vi "SetQuestionableInstrumentSMURegister.vi"(7 "SMU":T2, 8 "Error In":errorcluster, 9 "Questionable Instrument SMU Register":bool[](array[boolean])=[FALSE, FALSE, FALSE, FALSE, FALSE, FALSE, FALSE, FALSE, FALSE, FALSE, FALSE, FALSE, FALSE, FALSE, FALSE], 10 "Program Register":T1, 11 "Keithley 2602 In":refnum<visa-resource-name>) -> (0 "Error Out":errorcluster, 3 "Keithley 2602 Out":refnum<visa-resource-name>)   [LabVIEW 2012, in "Keithley-2602.lvlib"]
uses:
  Keithley-2602.lvlib
  Controls/SMU.ctl
  Controls/ProgramRegister.ctl
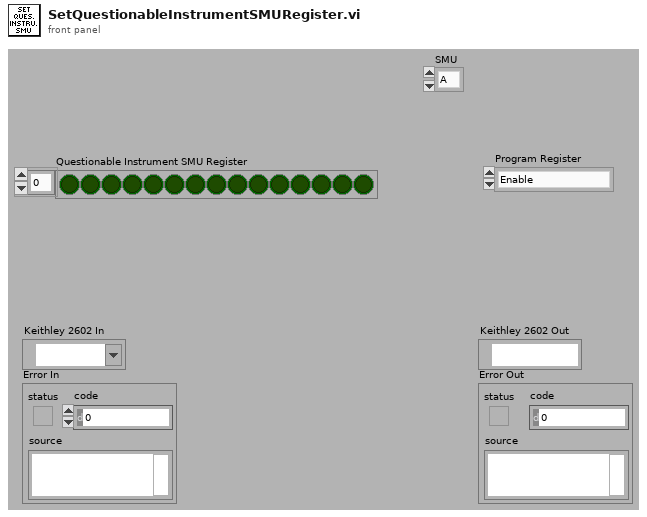
[diagram p1: front panel]
types:
  T1 = typedef "Keithley-2602.lvlib/ProgramRegister.ctl" = enum16{"Enable", "Positive Transition", "Negative Transition"}
  T2 = typedef "Keithley-2602.lvlib/SMU.ctl" = enum16{"A", "B"}
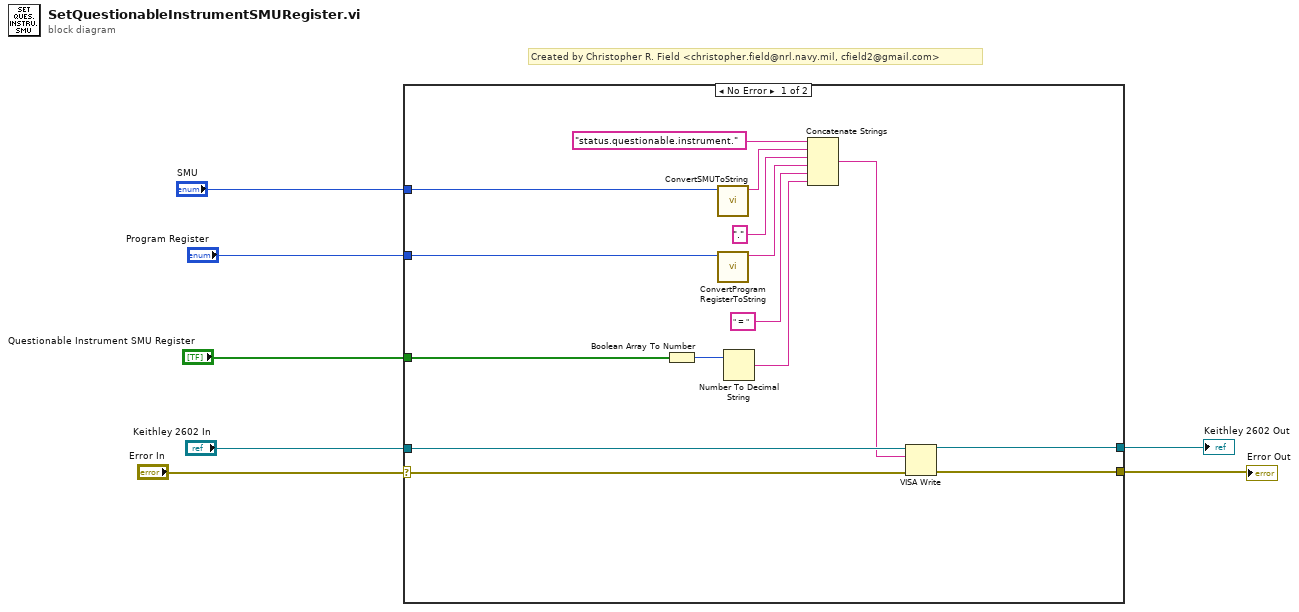
[diagram p0: block diagram]
diagram:
  # "Created by Christopher R. Field <christopher.field@nrl.navy.mil, cfield2@gmail.com>"
  n1 = case shown="No Error" "Error In" {
    selector: "Error In" -> [w8 w23]
    tunnel: "Keithley 2602 In" -> [w22 w24]
    tunnel: [w20 w24] -> w6
    tunnel: [w19 w23] -> w5
    tunnel: "Questionable Instrument SMU Register" -> [w18 _]
    tunnel: "Program Register" -> [w10 _]
    tunnel: "SMU" -> [w9 _]
    frame No Error {
      n2 = Boolean Array To Number(Boolean array=w18) -> (number=w21:u32)
      n3 = call "ConvertSMUToString.vi"("SMU"=w9) -> ("Channel"=w16:string)  [unwired: 10 in]
      n4 = call "ConvertProgramRegisterToString.vi"("Program Register"=w10) -> ("Register"=w14:string)  [unwired: 10 in]
      n5 = Number To Decimal String(number=w21) -> (decimal integer string=w12:string)  [unwired: 1 in]
      n6 = Concatenate Strings("status.questionable.instrument.", w16, "." ("string"), w14, " = " ("string"), w12) -> (w11:string)
      n7 = VISA Write(VISA resource name=w22, write buffer=w11, error in (no error)=w8) -> (VISA resource name out=w20:refnum<visa-resource-name>, error out=w19:errorcluster)  [unwired: 1 out]
    }
    frame Error {
    }
  }
  "Keithley 2602 Out" <- w6
  "Error Out" <- w5
